vi "Pc control.vi"() -> ()   [LabVIEW 2017]
uses:
  <vilib>/Utility/inputDevices.llb/joystickAcquire.vi
panel:
  out "Speed R":dbl
  out "Speed L":dbl
  in  "Speed Limit":dbl
  in  "stop":bool
  in  "error in (no error)":errorcluster
  out "Dir":bool
  out "error out":errorcluster
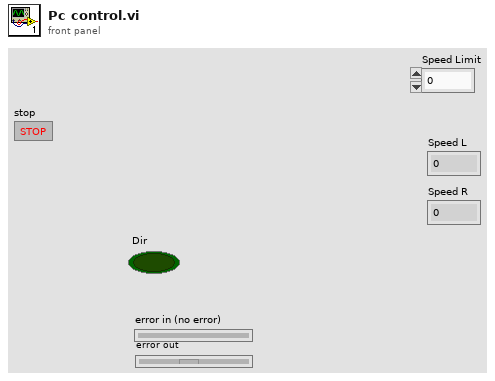
[diagram p1: front panel]
types:
  T1 = cluster{"X axis":i32, "Y axis":i32, "Z axis":i32, "X axis rotation":i32, "Y axis rotation":i32, "Z axis rotation":i32, "U axis":i32, "V axis":i32}
  T2 = cluster{"button 1":bool, "button 2":bool, "button 3":bool, "button 4":bool, "button 5":bool, "button 6":bool, "button 7":bool, "button 8":bool, "button 9":bool, "button 10":bool, "button 11":bool, "button 12":bool, "button 13":bool, "button 14":bool, "button 15":bool, "button 16":bool, "button 17":bool, "button 18":bool, "button 19":bool, "button 20":bool, "button 21":bool, "button 22":bool, "button 23":bool, "button 24":bool, "button 25":bool, "button 26":bool, "button 27":bool, "button 28":bool, "button 29":bool, "button 30":bool, "button 31":bool, "button 32":bool}
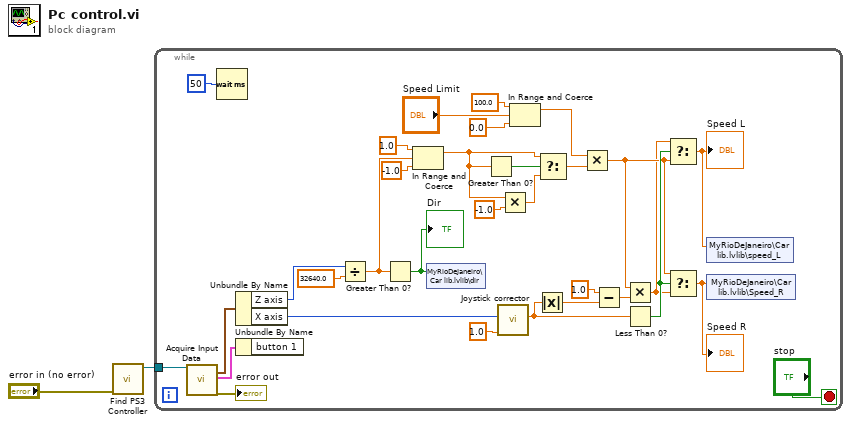
[diagram p0: block diagram]
diagram:
  n1 = call "Find PS3 Controller.vi"("error in (no error)"="error in (no error)") -> ("Controller Reference Out"=w1:refnum<k1>)  [unwired: 9 in, 1 out]
  n2 = while {
    tunnel: w1 -> [w31]
    stop <- "stop" stop-if-true
    n3 = call-poly <vilib>:"Acquire Input Data.vi"("device ID"=w31) -> ("axis info"=w32:T1, "button info"=w34:T2, "error out"=→"error out":errorcluster)  [unwired: 1 in, 15 out]
    n4 = Wait (ms)(milliseconds to wait=u32 50) -> ()  [unwired: 1 out]
    n5 = Unbundle By Name(w32) -> ("Z axis"=w24:i32, "X axis"=w28:i32)
    n6 = Unbundle By Name(w34) -> ()  [unwired: 1 out]
    n7 = Divide(x=w24, y=32640.0) -> (x/y=w14:dbl)
    n8 = Greater Than 0?(x=w14) -> (x > 0?=w3:bool)
    "Dir" <- w3
    n9 = In Range and Coerce(upper limit=1.0, x=w14, lower limit=-1.0) -> (coerced(x)=w17:dbl)  [unwired: 1 out]
    n10 = shared-variable "MyRioDeJaneiro\\Car lib.lvlib\\dir"(w3) -> ()  [unwired: 1 in, 1 out]
    n11 = Greater Than 0?(x=w17) -> (x > 0?=w19:bool)
    n12 = call "Joystick corrector.vi"("rate"=1.0, "Joystick"=w28) -> ("output"=w10:dbl)  [unwired: 9 in]
    n13 = Multiply(x=w17, y=-1.0) -> (x*y=w15:dbl)
    n14 = In Range and Coerce(upper limit=100.0, x="Speed Limit", lower limit=0.0) -> (coerced(x)=w20:dbl)  [unwired: 1 out]
    n15 = Absolute Value(x=w10) -> (abs(x)=w12:dbl)
    n16 = Select(t=w17, s=w19, f=w15) -> (s? t:f=w18:dbl)
    n17 = Multiply(x=w20, y=w18) -> (x*y=w7:dbl)
    n18 = Subtract(x=1.0, y=w12) -> (x-y=w8:dbl)
    n19 = Multiply(x=w7, y=w8) -> (x*y=w6:dbl)
    n20 = Less Than 0?(x=w10) -> (x < 0?=w9:bool)
    n21 = Select(t=w6, s=w9, f=w7) -> (s? t:f=w4:dbl)
    "Speed L" <- w4
    n22 = Select(t=w7, s=w9, f=w6) -> (s? t:f=w5:dbl)
    "Speed R" <- w5
    n23 = shared-variable "MyRioDeJaneiro\\Car lib.lvlib\\speed_L"(w4) -> ()  [unwired: 1 in, 1 out]
    n24 = shared-variable "MyRioDeJaneiro\\Car lib.lvlib\\Speed_R"(w5) -> ()  [unwired: 1 in, 1 out]
  }
